vi "Edge_Detection.vi"() -> ()   [LabVIEW 2025]
uses:
  <vilib>/vision/NI_Vision_Development_Module.lvlib
panel:
  out "File Type out":string
  out "Normal Edge":T1(plugin-control)
  out "Image":T1(plugin-control)
  in  "File Path":path
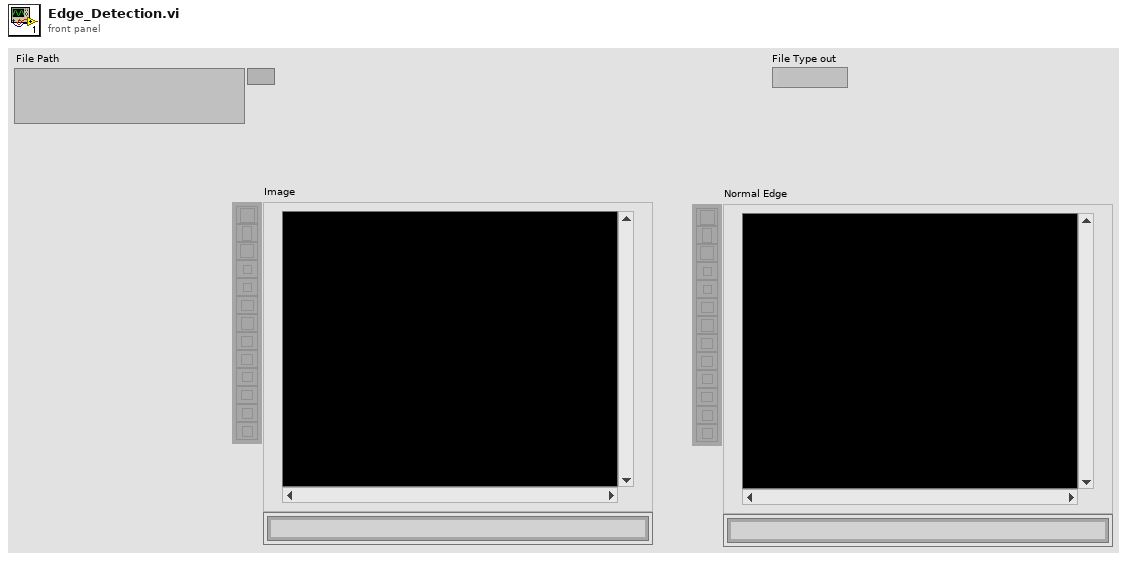
[diagram p1: front panel]
types:
  T1 = typedef "IMAQ Image.ctl" = refnum<image>
  T2 = enum32{"Differentiation", "Gradient", "Prewitt", "Roberts", "Sigma", "Sobel"}
  T3 = typedef "Image Type" = u32
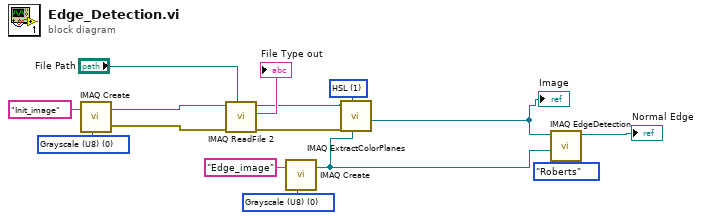
[diagram p0: block diagram]
diagram:
  w5 = u16 1 items=["RGB", "HSL", "HSV", "HSI"] ("Color Mode")
  w9 = T3 0 items=["Grayscale (U8)", "Grayscale (I16)", "Grayscale (SGL)", "Complex (CSG)", "RGB (U32)", "HSL (U32)", "RGB (U64)", "Grayscale (U16)"] ("Image Type")
  w13 = T3 0 items=["Grayscale (U8)", "Grayscale (I16)", "Grayscale (SGL)", "Complex (CSG)", "RGB (U32)", "HSL (U32)", "RGB (U64)", "Grayscale (U16)"] ("Image Type")
  n1 = call "IMAQ Create"("Image Name"="Init_image", "Image Type"=w13) -> ("New Image"=w14:T1, "error out"=w15:errorcluster)  [unwired: 3 in]
  n2 = call "IMAQ ReadFile 2"("File Path"="File Path", "error in (no error)"=w15, "Image"=w14) -> ("error out"=w3:errorcluster, "File Type out"=→"File Type out":string, "Image Out"=w2:T1)  [unwired: 4 in, 2 out]
  n3 = call "IMAQ Create"("Image Name"="Edge_image", "Image Type"=w9) -> ("New Image"=w1:T1)  [unwired: 3 in, 1 out]
  n4 = call "IMAQ ExtractColorPlanes"("Blue or Luma or Val or Inten Plane"=w1, "Color Mode"=w5, "error in (no error)"=w3, "Image Src"=w2) -> ("Blue or Luma or Val or Inten Plane out"=w4:T1)  [unwired: 4 in, 3 out]
  "Image" <- w4
  n5 = call "IMAQ EdgeDetection"("Method"=T2."Roberts", "Image Dst"=w1, "Image Src"=w4) -> ("Image Dst Out"=→"Normal Edge":T1)  [unwired: 7 in, 1 out]
